vi "SQL TESTING.vi"() -> ()   [LabVIEW 2017]
uses:
  <vilib>/addons/database/Connection.llb/Conn ObjectReference.ctl
  <vilib>/addons/database/Connection.llb/DB Tools Open Connec (Path).vi
  <vilib>/addons/database/Connection.llb/Conn Execute.vi
  <vilib>/addons/database/Recordset.llb/Rec Fetch Recordset Data (R).vi
  <vilib>/addons/database/Recordset.llb/Rec Destroy - Connection.vi
  <userlib>/_OpenG.lib/array/array.llb/Search 1D Array (String)__ogtk.vi
  <userlib>/_OpenG.lib/array/array.llb/Delete Elements from 1D Array (String)__ogtk.vi
  <vilib>/addons/database/NI_Database_API.lvlib
panel:
  out "element 6":string
  out "element 5":string
  out "Table 3":string[][](array[string])
  in  "error in (no error) 3":errorcluster
  out "error out 4":errorcluster
  out "connection reference 4":T1
  out "Production Count 3":i32
  out "size(s) 4":i32[](array[numeric])
  out "ACTUAL  PLC PRODUCT CODE 2":i32
  out "resulting string 3":string
  out "resulting string 2":string
  out "ACTUAL  PLC PRODUCT CODE":i32
  out "ACTUAL  PLC COUNT":i32
  out "size(s) 3":i32[](array[numeric])
  out "Production Count 2":i32
  out "connection reference 3":T1
  out "error out 3":errorcluster
  in  "error in (no error) 2":errorcluster
  out "Table 2":string[][](array[string])
  out "element 4":string
  out "element 3":string
  out "x = y?":bool
  out "size(s) 2":i32[](array[numeric])
  out "Production Count":i32
  out "connection reference 2":T1
  out "error out 2":errorcluster
  in  "error in (no error)":errorcluster
  out "Table":string[][](array[string])
  out "resulting string":string
  out "element 2":string
  out "element":string
  out "Shift":i32
  out "error out":errorcluster
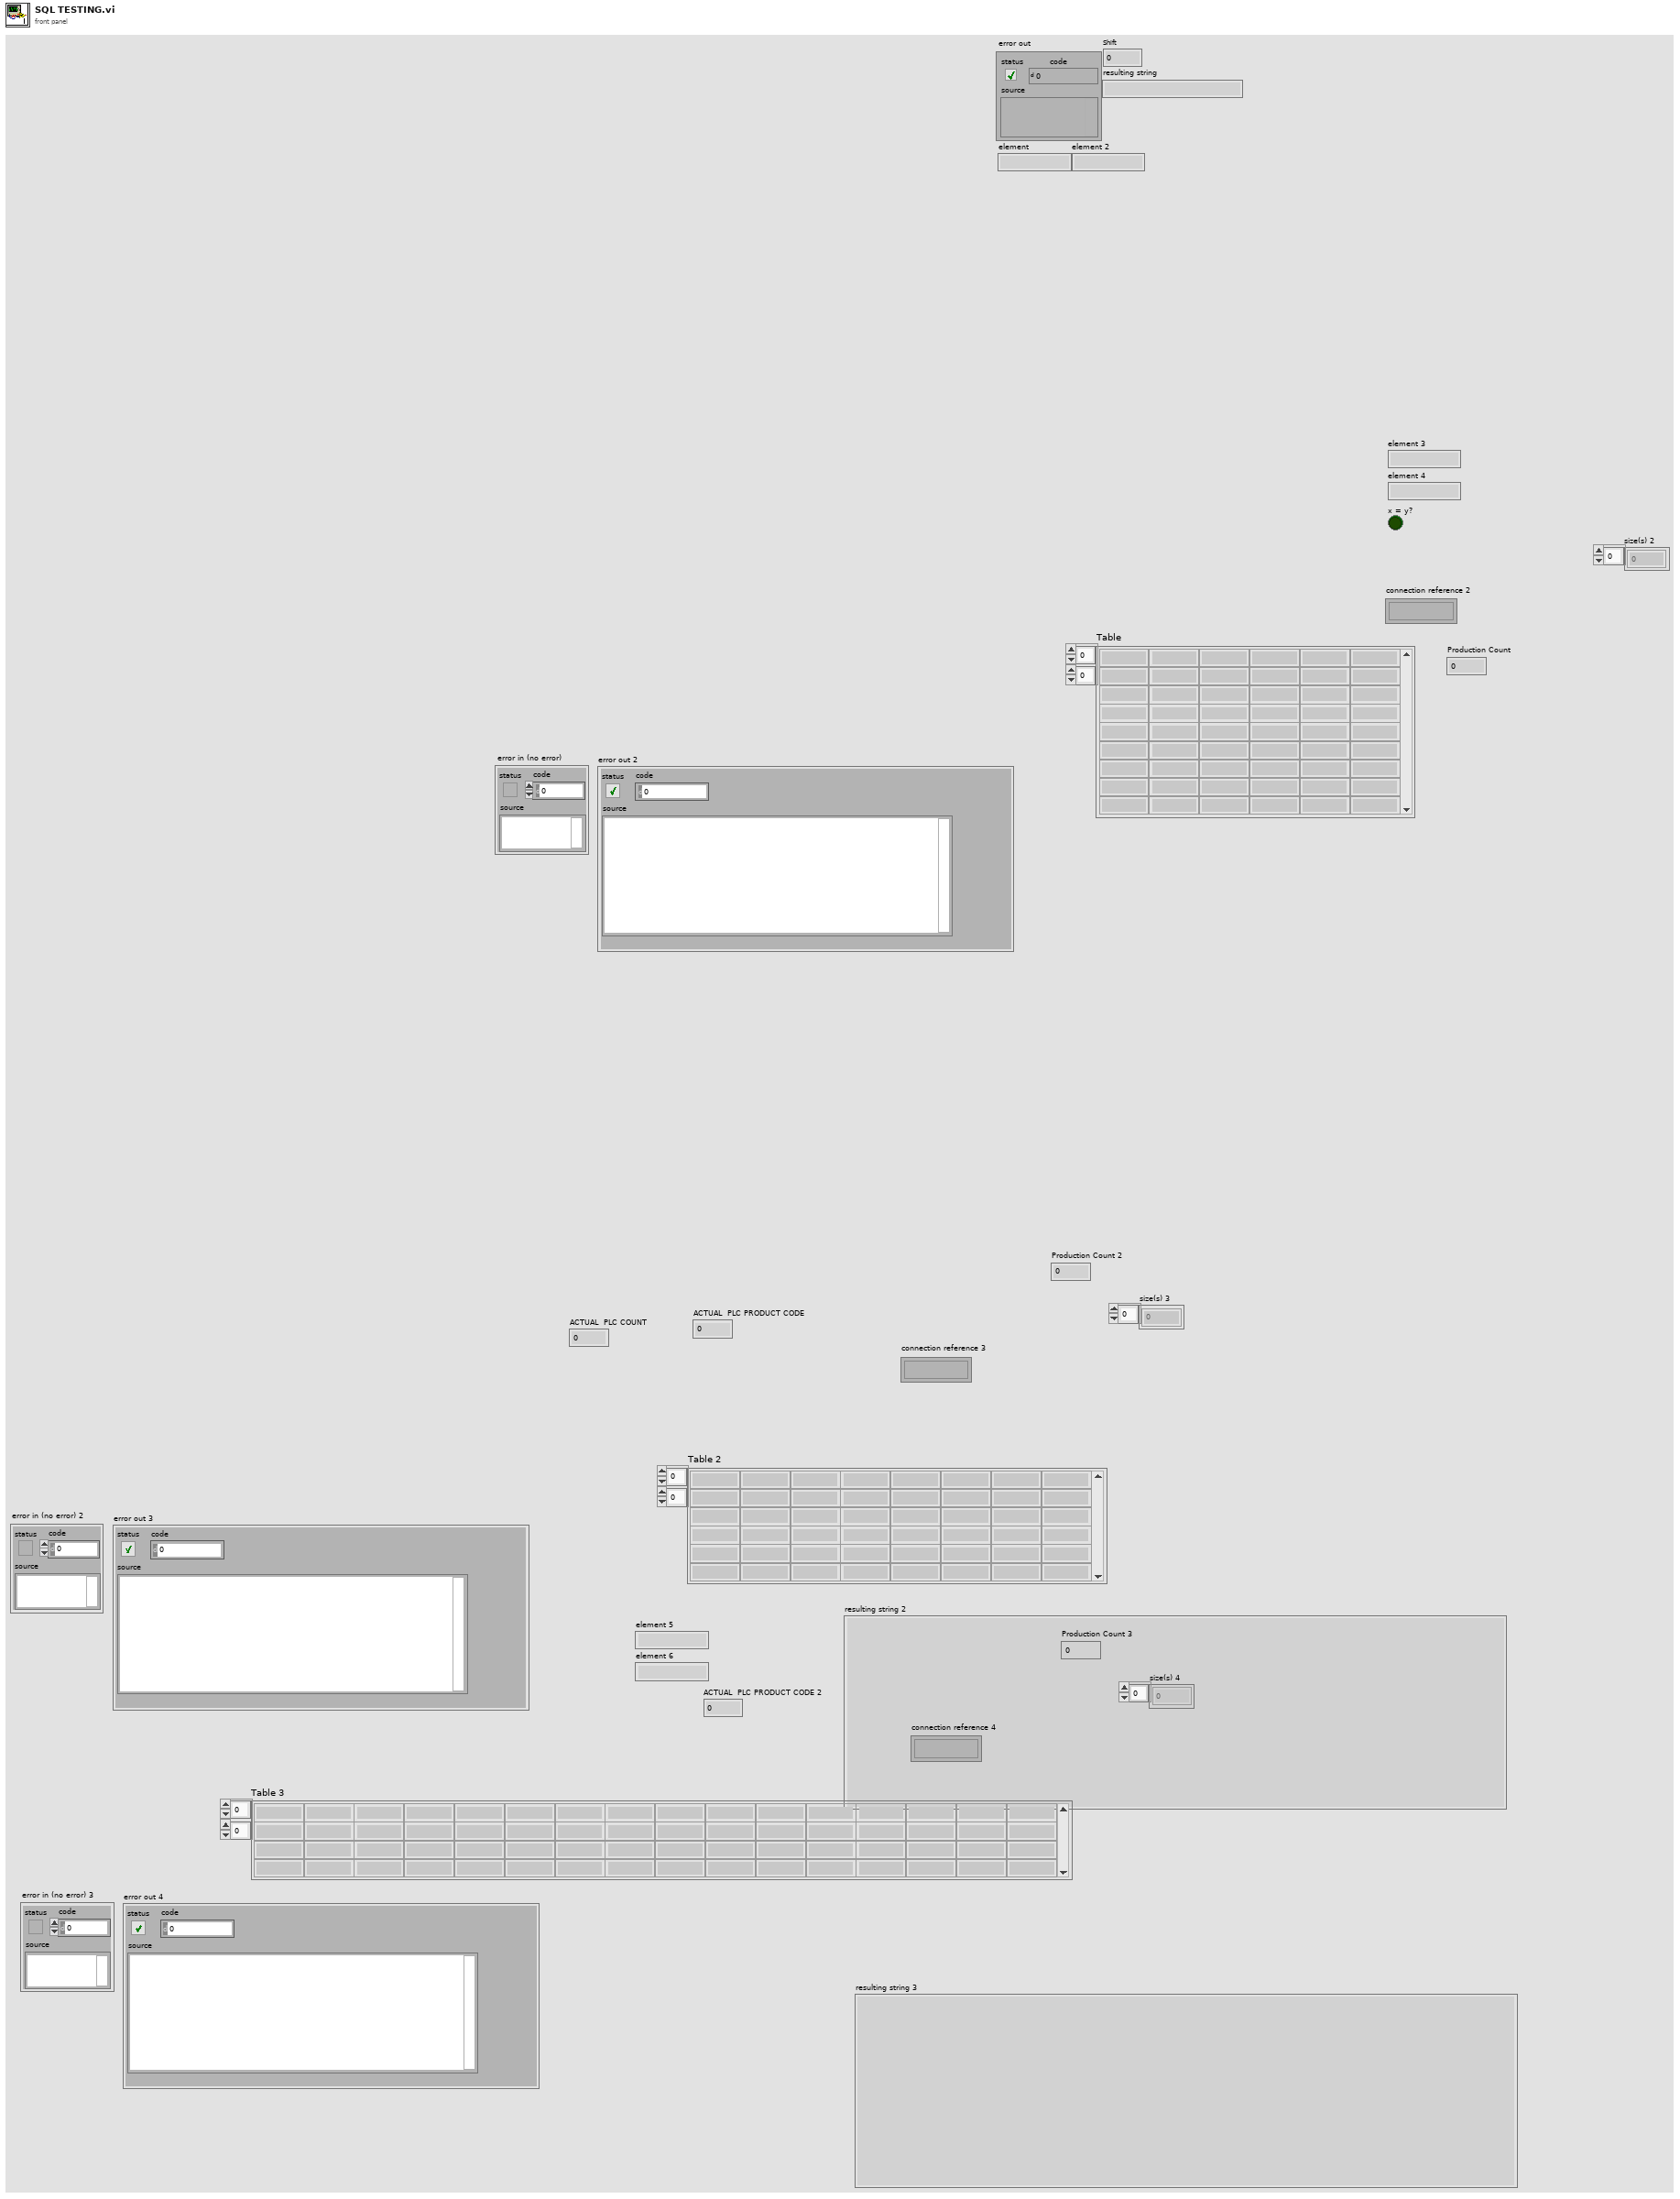
[diagram p1: front panel]
types:
  T1 = typedef "NI_Database_API.lvlib/Conn ObjectReference.ctl" = refnum<k1>
  T2 = typedef "NI_Database_API.lvlib/Rec ObjectReference.ctl" = refnum<k1>
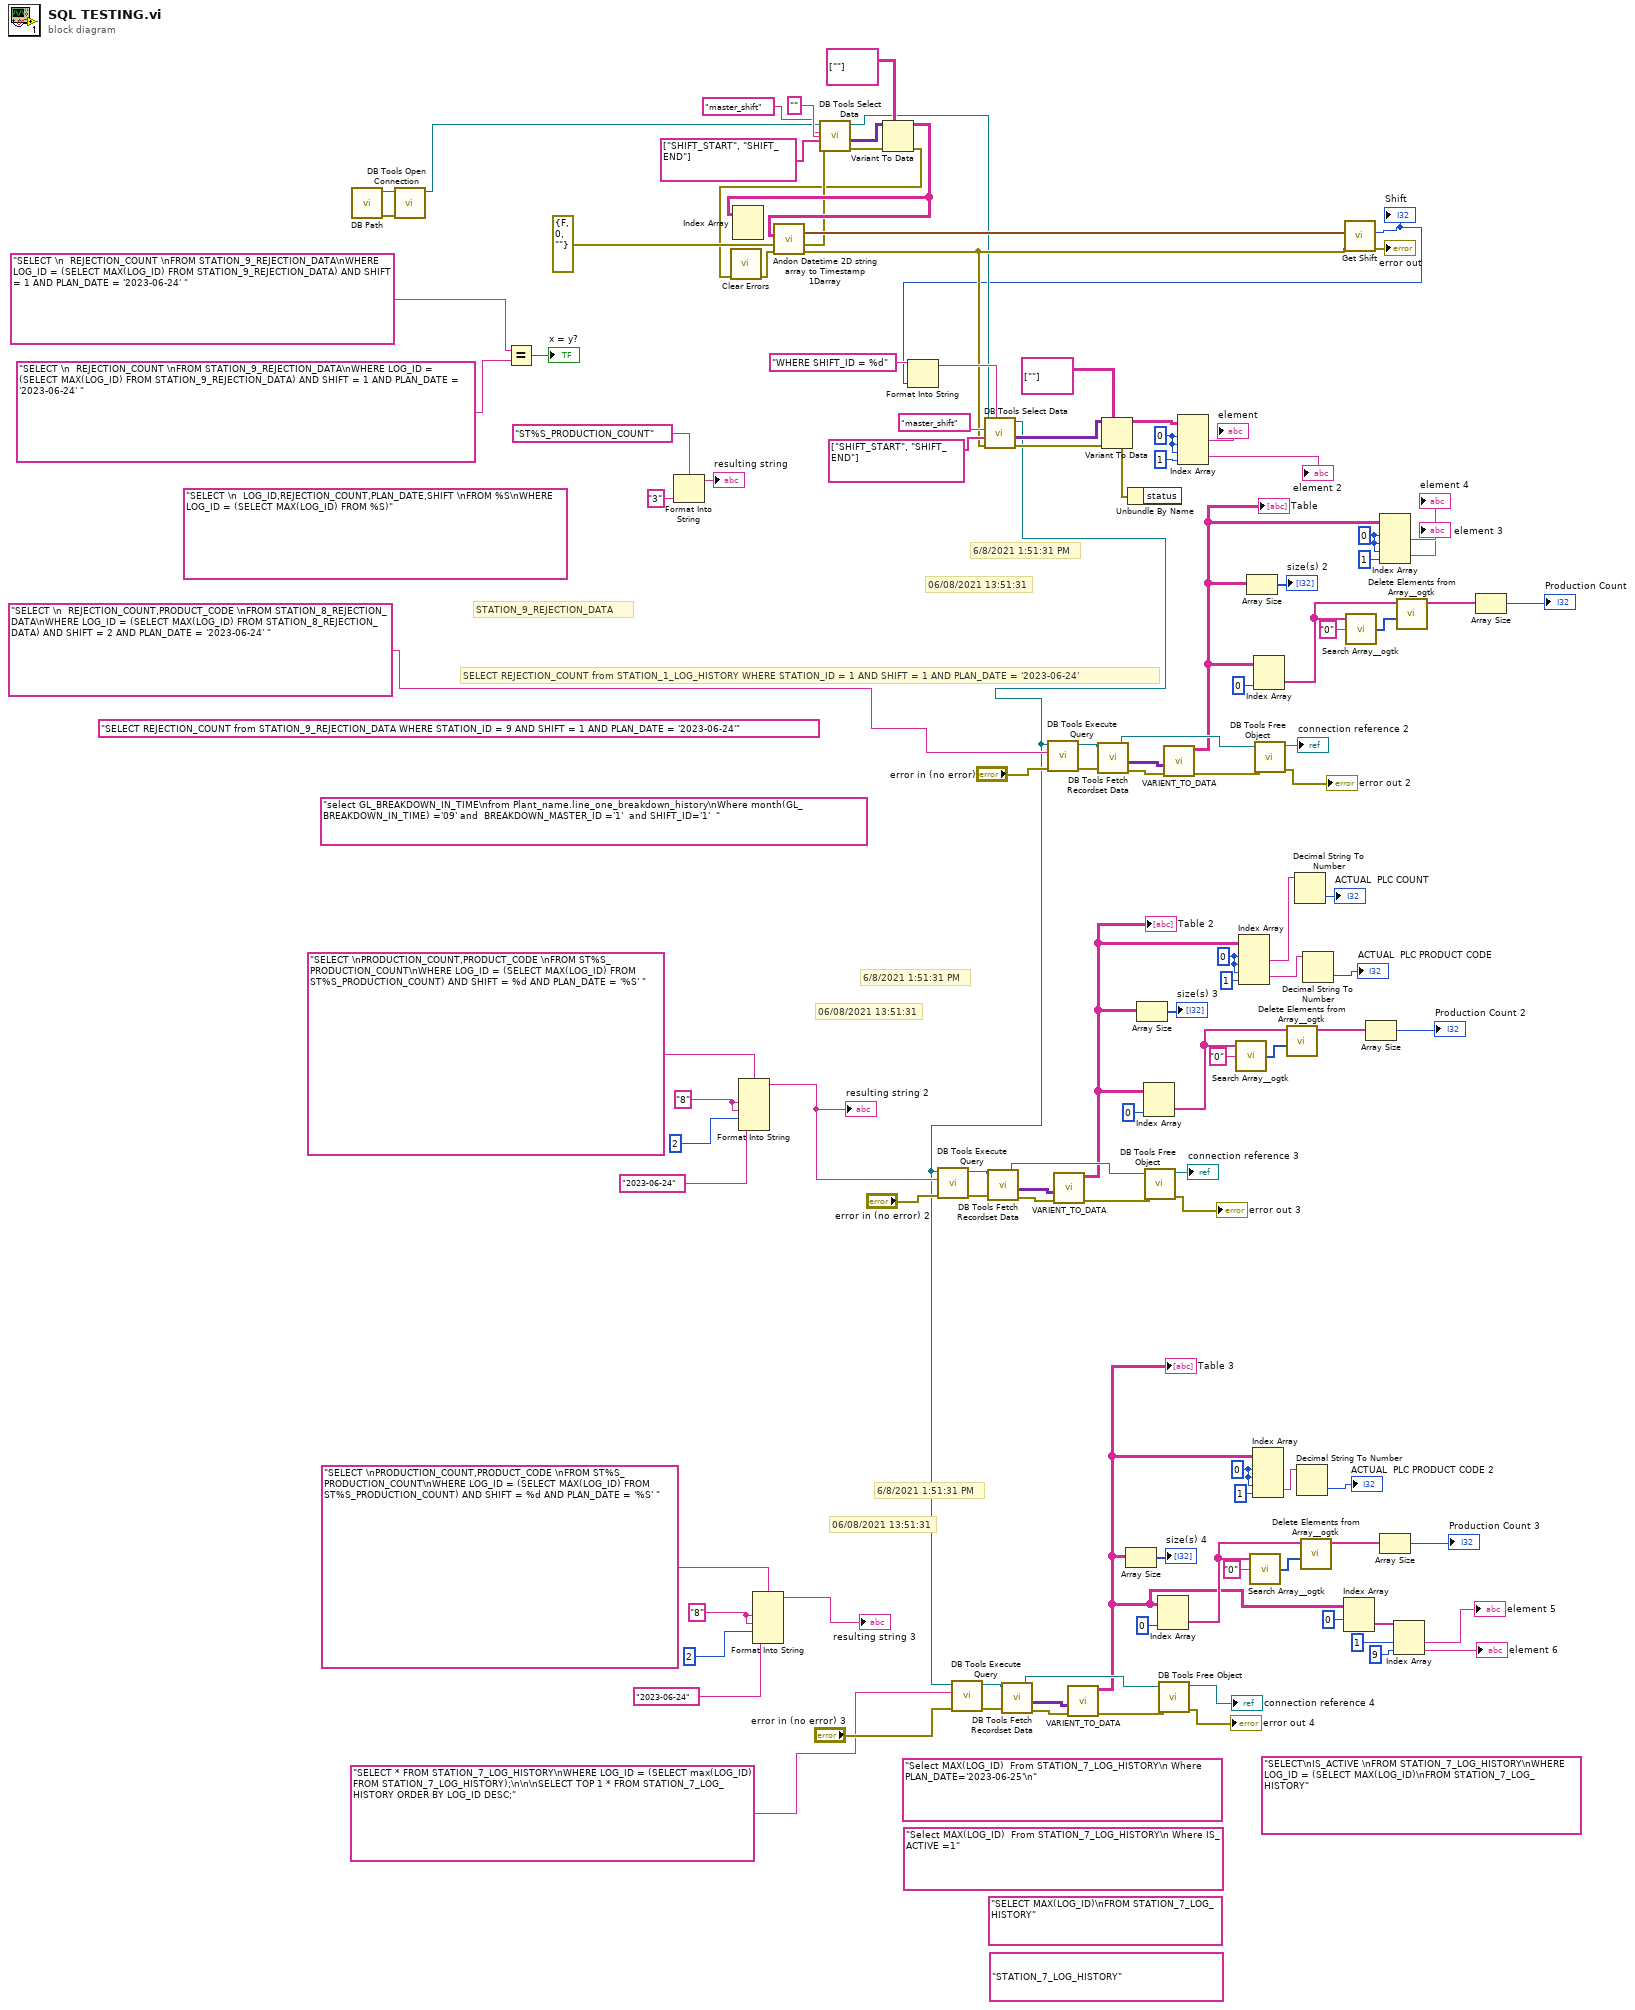
[diagram p0: block diagram]
diagram:
  (unwired) "SELECT MAX(LOG_ID)\nFROM STATION_7_LOG_HISTORY"
  (unwired) "SELECT\nIS_ACTIVE \nFROM STATION_7_LOG_HISTORY\nWHERE LOG_ID = (SELECT MAX(LOG_ID)\nFROM STATION_7_LOG_HISTORY"
  (unwired) "Select MAX(LOG_ID)  From STATION_7_LOG_HISTORY\n Where IS_ACTIVE =1"
  (unwired) "Select MAX(LOG_ID)  From STATION_7_LOG_HISTORY\n Where PLAN_DATE='2023-06-25'\n"
  (unwired) "STATION_7_LOG_HISTORY"
  w32 = "8" ("input 1")
  w26 = 0 ("index (row)")
  w37 = "8" ("input 1")
  w43 = 0 ("index (row)")
  w66 = 0 ("index (row)")
  (unwired) "SELECT \n  LOG_ID,REJECTION_COUNT,PLAN_DATE,SHIFT \nFROM %S\nWHERE LOG_ID = (SELECT MAX(LOG_ID) FROM %S)" ("SQL query")
  (unwired) "select GL_BREAKDOWN_IN_TIME\nfrom Plant_name.line_one_breakdown_history\nWhere month(GL_BREAKDOWN_IN_TIME) ='09' and  BREAKDOWN_MASTER_ID ='1'  and SHIFT_ID='1'  " ("String")
  (unwired) "SELECT REJECTION_COUNT from STATION_9_REJECTION_DATA WHERE STATION_ID = 9 AND SHIFT = 1 AND PLAN_DATE = '2023-06-24'" ("String")
  w98 = 0 ("index (row)")
  # "06/08/2021 13:51:31"
  # "6/8/2021 1:51:31 PM"
  # "06/08/2021 13:51:31"
  # "6/8/2021 1:51:31 PM"
  # "STATION_9_REJECTION_DATA"
  # "06/08/2021 13:51:31"
  # "6/8/2021 1:51:31 PM"
  # "SELECT REJECTION_COUNT from STATION_1_LOG_HISTORY WHERE STATION_ID = 1 AND SHIFT = 1 AND PLAN_DATE = '2023-06-24'"
  n1 = call "DB Path.vi"() -> ("error out"=w108:errorcluster, "DB Path"=w109:path)  [unwired: 10 in]
  n2 = call-poly <vilib>:"DB Tools Open Connection.vi"("error in (no error)"=w108, "connection information"=w109) -> ("connection reference"=w107:T1)  [unwired: 6 in, 1 out]
  n3 = Equal?(x="SELECT \n  REJECTION_COUNT \nFROM STATION_9_REJECTION_DATA\nWHERE LOG_ID = (SELECT MAX(LOG_ID) FROM STATION_9_REJECTION_DATA) AND SHIFT = 1 AND PLAN_DATE = '2023-06-24' " ("SQL query"), y="SELECT \n  REJECTION_COUNT \nFROM STATION_9_REJECTION_DATA\nWHERE LOG_ID = (SELECT MAX(LOG_ID) FROM STATION_9_REJECTION_DATA) AND SHIFT = 1 AND PLAN_DATE = '2023-06-24' " ("SQL query")) -> (x = y?=→"x = y?":bool)
  n4 = Format Into String(format string="ST%S_PRODUCTION_COUNT" ("Table name"), "3" ("input 1")) -> (resulting string=→"resulting string":string)  [unwired: 2 in, 1 out]
  n5 = Format Into String(format string="SELECT \nPRODUCTION_COUNT,PRODUCT_CODE \nFROM ST%S_PRODUCTION_COUNT\nWHERE LOG_ID = (SELECT MAX(LOG_ID) FROM ST%S_PRODUCTION_COUNT) AND SHIFT = %d AND PLAN_DATE = '%S' " ("SQL query"), w37, w37, 2 ("input 3"), "2023-06-24" ("input 4")) -> (resulting string=w38:string)  [unwired: 2 in, 1 out]
  "resulting string 2" <- w38
  n6 = Format Into String(format string="SELECT \nPRODUCTION_COUNT,PRODUCT_CODE \nFROM ST%S_PRODUCTION_COUNT\nWHERE LOG_ID = (SELECT MAX(LOG_ID) FROM ST%S_PRODUCTION_COUNT) AND SHIFT = %d AND PLAN_DATE = '%S' " ("SQL query"), w32, w32, 2 ("input 3"), "2023-06-24" ("input 4")) -> (resulting string=→"resulting string 3":string)  [unwired: 2 in, 1 out]
  n7 = call <vilib>:"DB Tools Select Data.vi"("condition"="", "error in (no error)"=errorcluster {"status"=FALSE, "code"=0, "source"=""}, "columns"=string[] ["SHIFT_START", "SHIFT_END"], "table"="master_shift", "connection reference"=w107) -> ("error out"=w120:errorcluster, "data"=w118:variant[][], "connection reference out"=w94:T1)  [unwired: 1 in]
  n8 = Variant To Data(error in=w120, type=string[][] [[""]], Variant=w118) -> (data=w119:string[][], error out=w110:errorcluster)
  n9 = call <vilib>:"Clear Errors.vi"("error in (no error)"=w110) -> ("error out"=w121:errorcluster)  [unwired: 5 in, 1 out]
  n10 = Index Array(array=w119) -> ()  [unwired: 2 in, 1 out]
  n11 = call "Andon Datetime 2D string array to Timestamp 1Darray.vi"("error in (no error)"=w121, "String Array In"=w119) -> ("error out"=w95:errorcluster, "Time Stamp Out"=w113:timestamp[])  [unwired: 8 in]
  n12 = call "Get Shift.vi"("error in (no error)"=w95, "Time Stamp Out"=w113) -> ("error out"=→"error out":errorcluster, "Shift"=w91:i32)  [unwired: 8 in]
  "Shift" <- w91
  n13 = Format Into String(format string="WHERE SHIFT_ID = %d", w91) -> (resulting string=w103:string)  [unwired: 2 in, 1 out]
  n14 = call <vilib>:"DB Tools Select Data.vi"("condition"=w103, "error in (no error)"=w95, "columns"=string[] ["SHIFT_START", "SHIFT_END"], "table"="master_shift", "connection reference"=w94) -> ("error out"=w101:errorcluster, "data"=w102:variant[][], "connection reference out"=w10:T1)  [unwired: 1 in]
  n15 = call-poly <vilib>:"DB Tools Execute Query.vi"("error in (no error)"="error in (no error) 2", "SQL query"=w38, "connection reference"=w10) -> ("error out"=w62:errorcluster, "recordset reference"=w59:T2)  [unwired: 5 in]
  n16 = call-poly <vilib>:"DB Tools Execute Query.vi"("error in (no error)"="error in (no error) 3", "SQL query"="SELECT * FROM STATION_7_LOG_HISTORY\nWHERE LOG_ID = (SELECT max(LOG_ID) FROM STATION_7_LOG_HISTORY);\n\n\nSELECT TOP 1 * FROM STATION_7_LOG_HISTORY ORDER BY LOG_ID DESC;", "connection reference"=w10) -> ("error out"=w11:errorcluster, "recordset reference"=w14:T2)  [unwired: 5 in]
  n17 = call-poly <vilib>:"DB Tools Fetch Recordset Data.vi"("error in (no error)"=w62, "recordset reference"=w59) -> ("error out"=w61:errorcluster, "recordset data"=w54:variant[][], "recordset reference out"=w58:T2)  [unwired: 3 in]
  n18 = call-poly <vilib>:"DB Tools Fetch Recordset Data.vi"("error in (no error)"=w11, "recordset reference"=w14) -> ("error out"=w12:errorcluster, "recordset data"=w19:variant[][], "recordset reference out"=w15:T2)  [unwired: 3 in]
  n19 = call-poly <vilib>:"DB Tools Execute Query.vi"("error in (no error)"="error in (no error)", "SQL query"="SELECT \n  REJECTION_COUNT,PRODUCT_CODE \nFROM STATION_8_REJECTION_DATA\nWHERE LOG_ID = (SELECT MAX(LOG_ID) FROM STATION_8_REJECTION_DATA) AND SHIFT = 2 AND PLAN_DATE = '2023-06-24' ", "connection reference"=w10) -> ("error out"=w87:errorcluster, "recordset reference"=w84:T2)  [unwired: 5 in]
  n20 = call "VARIENT_TO_DATA.vi"("data"=w54, "error in (no error)"=w61) -> ("Table"=w46:string[][], "error out"=w57:errorcluster)  [unwired: 7 in]
  "Table 2" <- w46
  n21 = call "VARIENT_TO_DATA.vi"("data"=w19, "error in (no error)"=w12) -> ("Table"=w7:string[][], "error out"=w16:errorcluster)  [unwired: 7 in]
  "Table 3" <- w7
  n22 = call-poly <vilib>:"DB Tools Fetch Recordset Data.vi"("error in (no error)"=w87, "recordset reference"=w84) -> ("error out"=w86:errorcluster, "recordset data"=w79:variant[][], "recordset reference out"=w83:T2)  [unwired: 3 in]
  n23 = Variant To Data(error in=w101, type=string[][] [[""]], Variant=w102) -> (data=w99:string[][], error out=w96:errorcluster)
  n24 = Array Size(array=w7) -> (size(s)=→"size(s) 4":i32[])
  n25 = Unbundle By Name(w96) -> ()  [unwired: 1 out]
  n26 = Array Size(array=w46) -> (size(s)=→"size(s) 3":i32[])
  n27 = Index Array(array=w46, index (col)=0 ("disabled index (col)")) -> (element=w50:string[])  [unwired: 1 in]
  n28 = call-poly <vilib>:"DB Tools Free Object.vi"("error in (no error)"=w57, "recordset reference"=w58) -> ("error out"=→"error out 3":errorcluster, "connection reference"=→"connection reference 3":T1)  [unwired: 8 in]
  n29 = Index Array(array=w7, index (col)=0 ("disabled index (col)")) -> (element=w8:string[])  [unwired: 1 in]
  n30 = call-poly <vilib>:"DB Tools Free Object.vi"("error in (no error)"=w16, "recordset reference"=w15) -> ("error out"=→"error out 4":errorcluster, "connection reference"=→"connection reference 4":T1)  [unwired: 8 in]
  n31 = call "VARIENT_TO_DATA.vi"("data"=w79, "error in (no error)"=w86) -> ("Table"=w67:string[][], "error out"=w82:errorcluster)  [unwired: 7 in]
  "Table" <- w67
  n32 = Index Array(array=w99, index (row) #1=w98, index (col) #1=w98, index (row) #2=w98, index (col) #2=1 ("disabled index (col)")) -> (element #1=→"element":string, element #2=→"element 2":string)
  n33 = call-poly <userlib>:"Search Array__ogtk.vi"("Array"=w50, "Element Data"="0") -> ("Indices of Elements"=w48:i32[])  [unwired: 7 in]
  n34 = Index Array(array=w46, index (row) #1=w43, index (col) #1=w43, index (row) #2=w43, index (col) #2=1 ("disabled index (col)")) -> (element #1=w45:string, element #2=w41:string)
  n35 = Array Size(array=w67) -> (size(s)=→"size(s) 2":i32[])
  n36 = call-poly <userlib>:"Search Array__ogtk.vi"("Array"=w8, "Element Data"="0") -> ("Indices of Elements"=w24:i32[])  [unwired: 7 in]
  n37 = Index Array(array=w7, index (row) #1=w26, index (col) #1=w26, index (row) #2=w26, index (col) #2=1 ("disabled index (col)")) -> (element #2=w28:string)  [unwired: 1 out]
  n38 = Index Array(array=w67, index (col)=0 ("disabled index (col)")) -> (element=w75:string[])  [unwired: 1 in]
  n39 = call-poly <vilib>:"DB Tools Free Object.vi"("error in (no error)"=w82, "recordset reference"=w83) -> ("error out"=→"error out 2":errorcluster, "connection reference"=→"connection reference 2":T1)  [unwired: 8 in]
  n40 = call-poly <userlib>:"Delete Elements from Array__ogtk.vi"("indices"=w48, "array"=w50) -> ("array w/ subset deleted"=w47:string[])  [unwired: 8 in, 1 out]
  n41 = Decimal String To Number(string=w45) -> (number=→"ACTUAL  PLC COUNT":i32)  [unwired: 2 in, 1 out]
  n42 = Decimal String To Number(string=w28) -> (number=→"ACTUAL  PLC PRODUCT CODE 2":i32)  [unwired: 2 in, 1 out]
  n43 = call-poly <userlib>:"Delete Elements from Array__ogtk.vi"("indices"=w24, "array"=w8) -> ("array w/ subset deleted"=w25:string[])  [unwired: 8 in, 1 out]
  n44 = Decimal String To Number(string=w41) -> (number=→"ACTUAL  PLC PRODUCT CODE":i32)  [unwired: 2 in, 1 out]
  n45 = Index Array(array=w7, index (row)=0) -> (element=w4:string[])  [unwired: 1 in]
  n46 = call-poly <userlib>:"Search Array__ogtk.vi"("Array"=w75, "Element Data"="0") -> ("Indices of Elements"=w73:i32[])  [unwired: 7 in]
  n47 = Array Size(array=w47) -> (size(s)=→"Production Count 2":i32)
  n48 = Index Array(array=w67, index (row) #1=w66, index (col) #1=w66, index (row) #2=w66, index (col) #2=1 ("disabled index (col)")) -> (element #1=→"element 3":string, element #2=→"element 4":string)
  n49 = Array Size(array=w25) -> (size(s)=→"Production Count 3":i32)
  n50 = Index Array(array=w4, index #1=1 ("index (row)"), index #2=9 ("index (row)")) -> (element #1=→"element 5":string, element #2=→"element 6":string)
  n51 = call-poly <userlib>:"Delete Elements from Array__ogtk.vi"("indices"=w73, "array"=w75) -> ("array w/ subset deleted"=w72:string[])  [unwired: 8 in, 1 out]
  n52 = Array Size(array=w72) -> (size(s)=→"Production Count":i32)
